vi "Write Payload .vi"(8 "error in (no error)":errorcluster, 10 "Payload":string, 11 "DataPacket in":refnum<class "DataPacket.lvclass">) -> (0 "error out":errorcluster, 3 "DataPacket out":refnum<class "DataPacket.lvclass">)   [LabVIEW 2021, in "DataPacket.lvclass"]
uses:
  DataPacket.lvclass
  DataPacket.lvclass/DataPacket.ctl
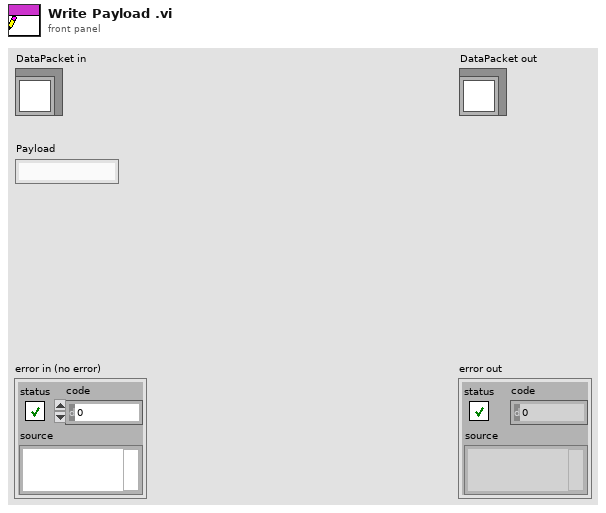
[diagram p1: front panel]
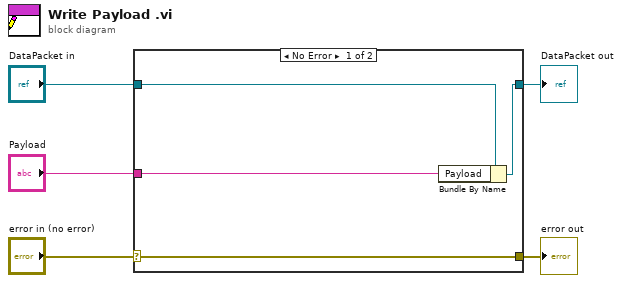
[diagram p0: block diagram]
diagram:
  n1 = case shown="No Error" "error in (no error)" {
    selector: "error in (no error)" -> [w9 w10]
    tunnel: [w9 w10] -> w4
    tunnel: [w7 w11] -> w2
    tunnel: "DataPacket in" -> [w8 w11]
    tunnel: "Payload" -> [w6 _]
    frame No Error {
      n2 = Bundle By Name(cluster=w8, "Payload"=w6) -> (w7:refnum<class "DataPacket.lvclass">)
    }
    frame Error {
    }
  }
  "error out" <- w4
  "DataPacket out" <- w2
